vi "Update Channel Value.vi"(8 "error in (no error)":errorcluster, 9 "New Value":dbl, 10 "Channel Index":i32, 11 "Output Process in":refnum<class "Sine Process.lvclass">) -> (0 "error out":errorcluster, 1 "# elements":u32, 2 "timed out?":bool, 3 "Output Process out":refnum<class "Sine Process.lvclass">)   [LabVIEW 2019, in "TimingDRV Engine.lvlib" / "Sine Process.lvclass"]
uses:
  Sine Process.lvclass
  Sine Process.lvclass/Sine Process.ctl
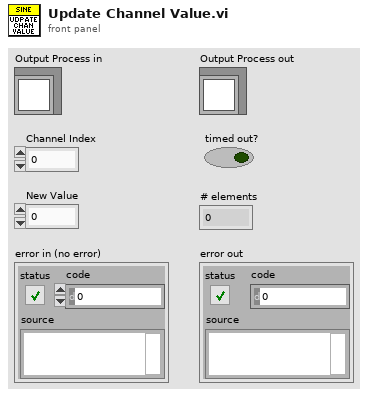
[diagram p1: front panel]
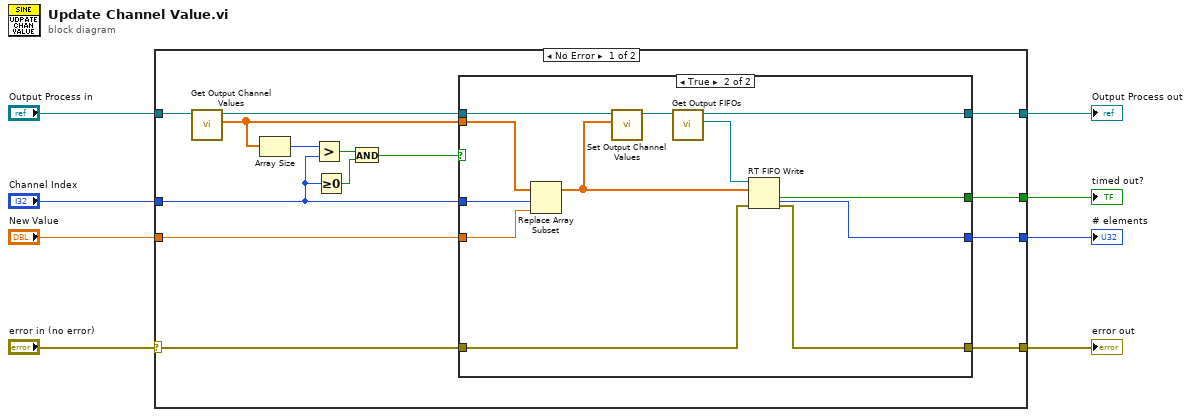
[diagram p0: block diagram]
diagram:
  n1 = case shown="No Error" "error in (no error)" {
    selector: "error in (no error)" -> [w15 w38]
    tunnel: [w22 w37] -> w8
    tunnel: [w21 _] -> w7
    tunnel: [w20 _] -> w6
    tunnel: [w19 w38] -> w5
    tunnel: "New Value" -> [w17 _]
    tunnel: "Channel Index" -> [w12 _]
    tunnel: "Output Process in" -> [w16 w37]
    frame No Error {
      n2 = call "Get Output Channel Values.vi"("Output Process in"=w16) -> ("Output Channel Values"=w14:dbl[], "Output Process out"=w18:refnum<class "Sine Process.lvclass">)  [unwired: 9 in]
      n3 = Array Size(array=w14) -> (size(s)=w13:i32)
      n4 = Greater?(x=w13, y=w12) -> (0:w11:bool)
      n5 = Greater Or Equal To 0?(x=w12) -> (x >= 0?=w10:bool)
      n6 = And(x=w11, y=w10) -> (x .and. y?=w9:bool)
      n7 = case shown="True" w9 {
        tunnel: [w24 w36] -> w22
        tunnel: [_ w35] -> w21
        tunnel: [_ w34] -> w20
        tunnel: [w23 w25] -> w19
        tunnel: w18 -> [w24 w30]
        tunnel: w17 -> [_ w29]
        tunnel: w15 -> [w23 w28]
        tunnel: w14 -> [_ w27]
        tunnel: w12 -> [_ w26]
        frame False {
        }
        frame True {
          n8 = Replace Array Subset(array=w27, new element=w29, index=w26) -> (w33:dbl[])
          n9 = call "Set Output Channel Values.vi"("Output Channel Values"=w33, "Output Process in"=w30) -> ("Output Process out"=w31:refnum<class "Sine Process.lvclass">)  [unwired: 9 in]
          n10 = call "Get Output FIFOs.vi"("Output Process in"=w31) -> ("Output FIFOs"=w32:refnum<k33>, "Output Process out"=w36:refnum<class "Sine Process.lvclass">)  [unwired: 9 in]
          n11 = RT FIFO Write(0:w32, 1:w33, 3:w28) -> (7:w35:u32, 10:w34:bool, 11:w25:errorcluster)  [unwired: 2 in, 1 out]
        }
      }
    }
    frame Error {
    }
  }
  "Output Process out" <- w8
  "# elements" <- w7
  "timed out?" <- w6
  "error out" <- w5
